vi "Load Step Classes.vi"(8 "error in (no error)":errorcluster, 11 "Step Classes Folder Path":path) -> (0 "error out":errorcluster, 3 "Step Class Library":T1)   [LabVIEW 2015, in "Configuration Tool.lvlib"]
uses:
  Configuration Tool.lvlib
  Controls/StepClassLibrary.ctl
  Prototype/classes/Step/Config/Step Config.lvclass
  Prototype/classes/Step/UI/Step UI.lvclass
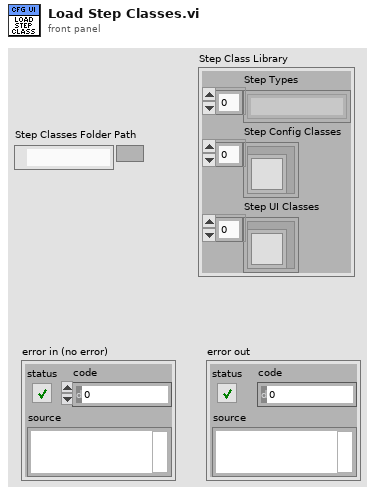
[diagram p1: front panel]
types:
  T1 = typedef "Configuration Tool.lvlib/StepClassLibrary.ctl" = cluster{"Step Types":string[], "Step Config Classes":refnum<class "Step Config.lvclass">[], "Step UI Classes":refnum<class "Step UI.lvclass">[]}
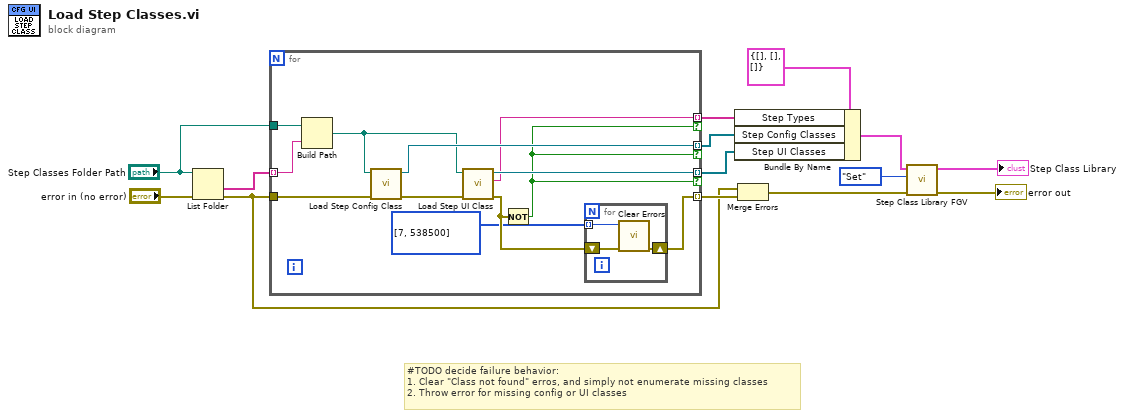
[diagram p0: block diagram]
diagram:
  # "#TODO decide failure behavior:\n1. Clear \"Class not found\" erros, and simply not enumerate missing classes\n2. Throw error for missing config or UI classes"
  n1 = List Folder(path="Step Classes Folder Path", error in="error in (no error)") -> (folder names=w1:string[], error out=w11:errorcluster)  [unwired: 2 in, 2 out]
  n2 = for {
    tunnel: [w22] -> w9 mode=indexing if=w18
    tunnel: w1 -> [w24] mode=indexing
    tunnel: "Step Classes Folder Path" -> [w25]
    tunnel: w11 -> [w26]
    tunnel: [w17] -> w14 mode=indexing
    tunnel: [w16] -> w2 mode=indexing if=w18
    tunnel: [w19] -> w3 mode=indexing if=w18
    n3 = Build Path(base path=w25, name or relative path=w24) -> (appended path=w20:path)
    n4 = call "Load Step Config Class.vi"("error in (no error)"=w26, "Step Folder Path"=w20) -> ("error out"=w23:errorcluster, "Step Config out"=w22:refnum<class "Step Config.lvclass">)  [unwired: 8 in]
    n5 = call "Load Step UI Class.vi"("error in (no error)"=w23, "Step Folder Path"=w20) -> ("error out"=w21:errorcluster, "Step Name"=w16:string, "Step UI out"=w19:refnum<class "Step UI.lvclass">)  [unwired: 7 in]
    n6 = Not(x=w21) -> (.not. x?=w18:bool)
    n7 = for {
      shift-right: [w28] -> w17
      shift-left: w21 -> [w29]
      tunnel: i32[] [7, 538500] -> [w27] mode=indexing
      n8 = call <vilib>:"Clear Errors.vi"("error in (no error)"=w29, "specific error code to clear (0: all)"=w27) -> ("error out"=w28:errorcluster)  [unwired: 4 in, 1 out]
    }
  }
  n9 = Bundle By Name(cluster=T1 {"Step Types"=[], "Step Config Classes"=[], "Step UI Classes"=[]}, "Step Types"=w2, "Step Config Classes"=w9, "Step UI Classes"=w3) -> (w5:T1)
  n10 = Merge Errors(w11, w14) -> (w7:errorcluster)
  n11 = call "Step Class Library FGV.vi"("error in (no error)"=w7, "Action"=enum16{"Set", "Get"}."Set", "Step Type Class Library"=w5) -> ("error out"=→"error out":errorcluster, "Step Type Class Library out"=→"Step Class Library":T1)  [unwired: 7 in]
